vi "setUp.vi"(8 "error in (no error)":errorcluster, 11 "reference in":refnum<class "testcase-Broadcast Registry.lvclass">) -> (0 "error out":errorcluster, 3 "reference out":refnum<class "testcase-Broadcast Registry.lvclass">)   [LabVIEW 2017, in "testcase-Broadcast Registry.lvclass"]
doc: "setUp runs prior to the test method during test execution. Use this method to initialize any object data required by your tests."
uses:
  testcase-Broadcast Registry.lvclass
  C:/Program Files (x86)/National Instruments/LabVIEW 2017/vi.lib/addons/_JKI Toolkits/VI Tester/TestCase.llb/TestCase.lvclass
  testcase-Broadcast Registry.lvclass/testcase-Broadcast Registry.ctl
  <vilib>/addons/_JKI Toolkits/VI Tester/TestCase.llb/TestCase.lvclass
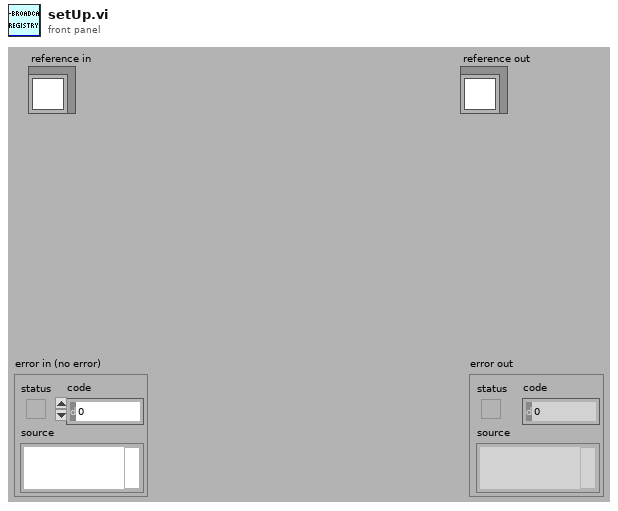
[diagram p1: front panel]
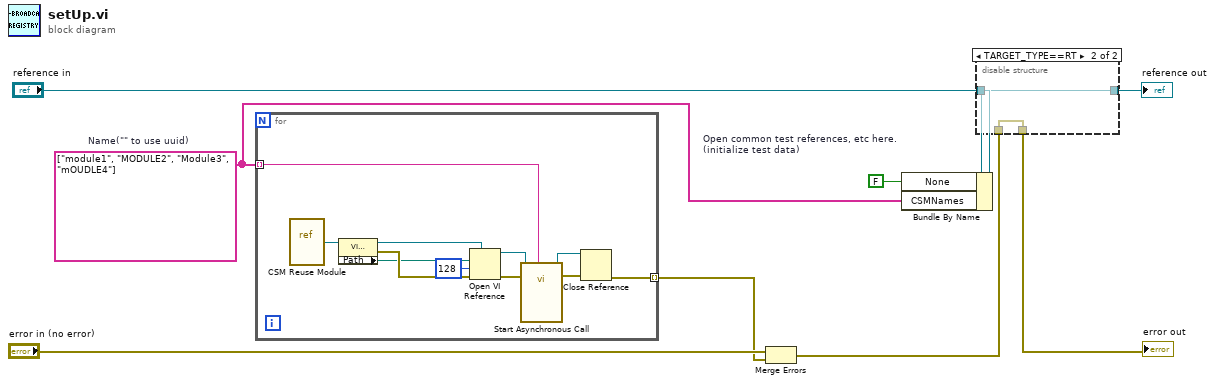
[diagram p0: block diagram]
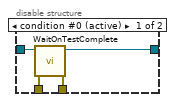
[diagram p2: hidden frame]
diagram:
  w1 = string[] ["module1", "MODULE2", "Module3", "mOUDLE4"]  # Name("" to use uuid)
  w4 = FALSE  # Open common test references, etc here. (initialize test data)
  n1 = for {
    tunnel: w1 -> [w17] mode=indexing
    tunnel: [w10] -> w2 mode=indexing
    n2 = vi-ref "CSM Reuse Module.vi"() -> (w12:refnum<vi>)
    n3 = property class="VI (strict)"(reference=w12) -> (reference out=w16:refnum<vi>, error out=w14:errorcluster, "Path"=w13:path)  [unwired: 1 in]
    n4 = Open VI Reference(type specifier VI Refnum (for type only)=w16, vi path=w13, options=128, error in (no error)=w14) -> (vi reference=w15:refnum<vi>, error out=w11:errorcluster)  [unwired: 2 in]
    n5 = call-by-ref "Start Asynchronous Call"(reference=w15, error in=w11, "Name(\"\" to use uuid)"=w17) -> (reference out=w19:refnum<vi>, error out=w18:errorcluster)  [unwired: 11 in]
    n6 = Close Reference(reference=w19, error in (no error)=w18) -> (error out=w10:errorcluster)
  }
  n7 = Merge Errors("error in (no error)", w2) -> (w3:errorcluster)
  n8 = Bundle By Name(cluster="reference in", "None"=w4, "CSMNames"=w1) -> (w5:refnum<class "testcase-Broadcast Registry.lvclass">)
  n9 = disable-structure shown="TARGET_TYPE==RT" {
    disable-tunnel: w3 -> [w24 w25]
    disable-tunnel: [w23 w25] -> w8
    disable-tunnel: [w22 w26] -> w6
    disable-tunnel: w5 -> [w21 w26]
    frame condition #0 (active) {
      n10 = call <vilib>:"WaitOnTestComplete.vi"("error in (no error)"=w24, "TestCase in"=w21) -> ("error out"=w23:errorcluster, "TestCase out"=w22:refnum<class "testcase-Broadcast Registry.lvclass">)  [unwired: 8 in]
    }
    frame condition #1 {
    }
  }
  "error out" <- w8
  "reference out" <- w6
